vi "Type.vi"(11 "GUI Element in":refnum<class "GUI Element.lvclass">) -> (2 "Element Type":string, 3 "GUI Element out":refnum<class "GUI Element.lvclass">)   [LabVIEW 2020, in "VolatusGUI.lvlib" / "GUI Element.lvclass"]
uses:
  GUI Element.lvclass
  GUI Element.lvclass/GUI Element.ctl
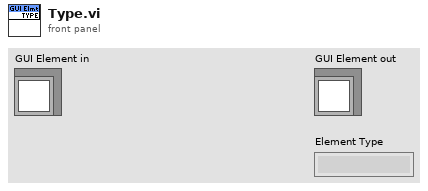
[diagram p1: front panel]
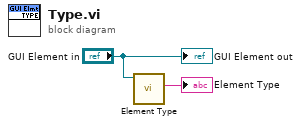
[diagram p0: block diagram]
diagram:
  n1 = call-dynamic "Element Type.vi"("GUI Element in"="GUI Element in") -> ("Element Type"=→"Element Type":string)  [unwired: 10 in]
  "GUI Element out" <- "GUI Element in"
